vi "Select Channel and Function.vi"(8 "error in (no error)":errorcluster, 10 "Channel":u16(ring) items=["A1"=0, "A2"=1, "A3"=2, "A4"=3, "A5"=4, "A6"=5, "A7"=6, "A8"=7, "A9"=8, "A10"=9, "K1"=200, "K2"=201, "K3"=202, "K4"=203, "FA1"=204, "FA2"=205, "FA3"=206, "FA4"=207], 11 "VISA resource name":refnum<visa-resource-name>) -> (0 "error out":errorcluster, 3 "VISA resource name out":refnum<visa-resource-name>)   [LabVIEW 2017, in "Sefram DAS220.lvlib"]
doc: "Select a channel from A1 to J20 (200 analog channels) and from K1 to K4 (digital function channels : PWM, Frequency, Counter). Function channel are accessible from FA1(204) to FJ4(243)."
uses:
  <instrlib>/Sefram DAS220/Sefram DAS220.lvlib
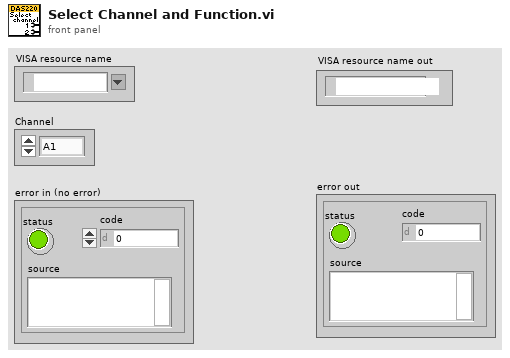
[diagram p1: front panel]
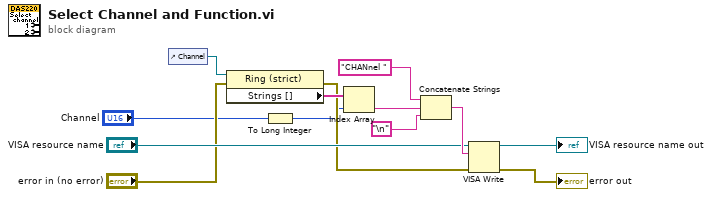
[diagram p0: block diagram]
diagram:
  n1 = control-ref of="Channel"() -> (w2:refnum<vi>)
  n2 = property class="Ring (strict)"(reference=w2, error in="error in (no error)") -> (error out=w4:errorcluster, "Strings []"=w9:string[])  [unwired: 1 out]
  n3 = To Long Integer(number="Channel") -> (32bit integer=w3:i32)
  n4 = Index Array(array=w9, index=w3) -> (element=w8:string)
  n5 = Concatenate Strings("CHANnel " ("string"), w8, "\n") -> (w12:string)
  n6 = VISA Write(VISA resource name="VISA resource name", write buffer=w12, error in (no error)=w4) -> (VISA resource name out=→"VISA resource name out":refnum<visa-resource-name>, error out=→"error out":errorcluster)  [unwired: 1 out]
